vi "getParameter_name.vi"(8 "error in (no error)":errorcluster, 11 "ScriptEvent in":refnum<class "ScriptEvent.lvclass">) -> (0 "error out":errorcluster, 2 "parameter_name":string, 3 "ScriptEvent out":refnum<class "ScriptEvent.lvclass">)   [LabVIEW 2011, in "Tools.lvlib" / "Scripting.lvlib" / "ScriptEvent.lvclass"]
uses:
  ScriptEvent.lvclass
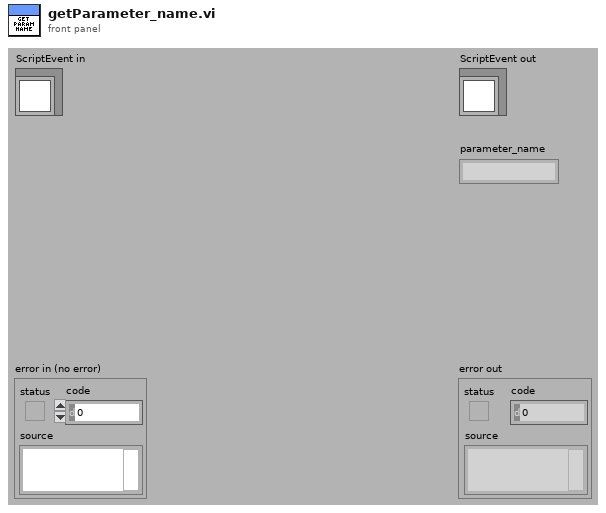
[diagram p1: front panel]
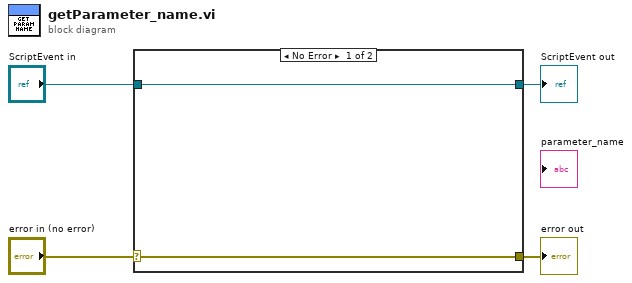
[diagram p0: block diagram]
diagram:
  n1 = case shown="No Error" "error in (no error)" {
    selector: "error in (no error)" -> [w6 w7]
    tunnel: [w6 w7] -> w3
    tunnel: [w5 w8] -> w1
    tunnel: "ScriptEvent in" -> [w5 w8]
    frame No Error {
    }
    frame Error {
    }
  }
  "error out" <- w3
  "ScriptEvent out" <- w1
